vi "LabVIEW to TOML.vi"(8 "error in (no error)":errorcluster, 11 "LV Value":variant) -> (0 "error out":errorcluster, 2 "Name":string, 3 "TOML Value":T1)   [LabVIEW 2020, in "TOML.lvlib"]
uses:
  TOML.lvlib
  TOML Value.ctl
  Value.ctl
  Value Type.ctl
  Key-Value Pair.ctl
  <vilib>/ErrorRing/Error Ring.xnode
  <vilib>/Utility/Data Type/NI_Data Type.lvlib
  <vilib>/JDP Science/JDP Science Common Utilities/JDP Utility.lvlib
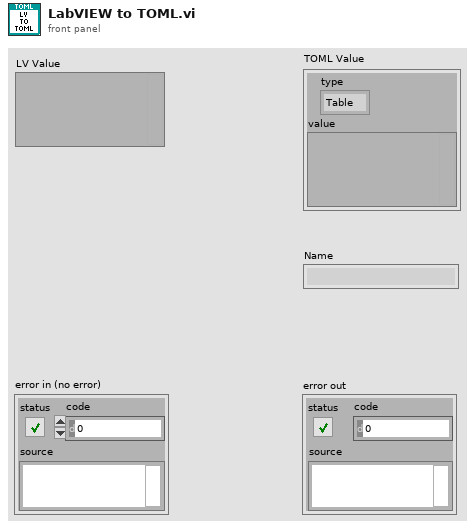
[diagram p1: front panel]
types:
  T1 = typedef "TOML.lvlib/TOML Value.ctl" = cluster{"type":enum16{"Table", "Array", "String", "Integer", "Float", "Boolean", "Offset Date-Time", "Local Date-Time", "Local Date", "Local Time", "Path"}, "value":variant}
  T2 = typedef "TOML.lvlib/Value.ctl" = cluster{"Type":T3, "Value":variant}
  T3 = typedef "TOML.lvlib/Value Type.ctl" = enum16{"Table", "Array", "String", "Integer", "Float", "Boolean", "Offset Date-Time", "Local Date-Time", "Local Date", "Local Time", "Path"}
  T4 = typedef "TOML.lvlib/Key-Value Pair.ctl" = cluster{"Key":string, "Value":T2}
  T5 = typedef "NI_Data Type.lvlib/Data Type.ctl" = enum8{"Invalid Type", "Void", "I8", "I16", "I32", "I64", "U8", "U16", "U32", "U64", "Single Float", "Double Float", "Extended Float", "Single Complex", "Double Complex", "Extended Complex", "Enum U8", "Enum U16", "Enum U32", "Enum U64", "Single Float With Unit", "Double Float With Unit", "Extended Float With Unit", "Single Complex with Unit", "Double Complex with Unit", "Extended Complex with Unit", "Boolean", "String", "Path", "Picture", "Tag", "Array", "Cluster", "Variant", "LV Variant", "Waveform", "Timestamp", "Digital Waveform", "Digital Data", "ExpressData", "Refnum", "External Data", "VI", "Poly VI", "LabVIEW Class Instance", "Fixed Point", "Set Collection", "Map Collection"}
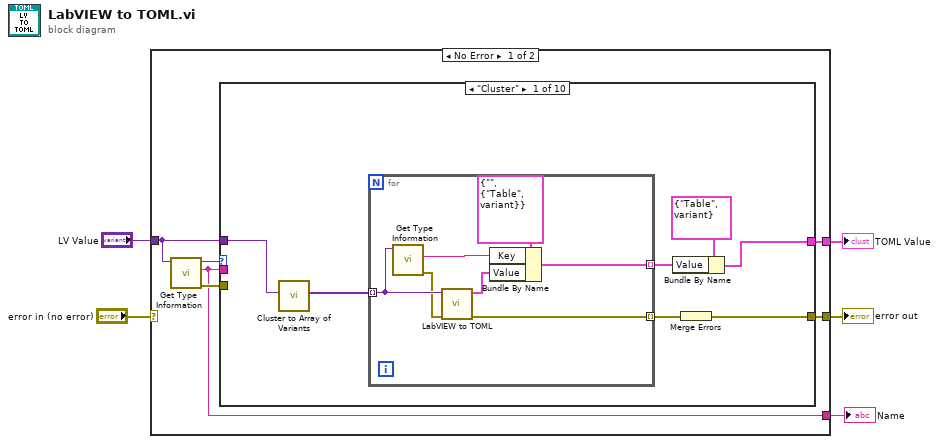
[diagram p0: block diagram]
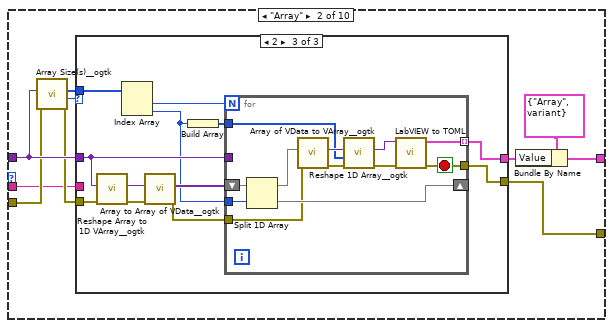
[diagram p2: hidden frame]
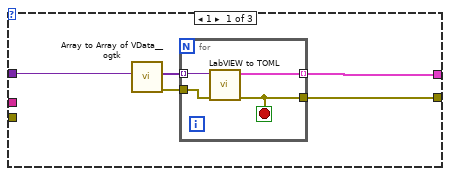
[diagram p3: hidden frame]
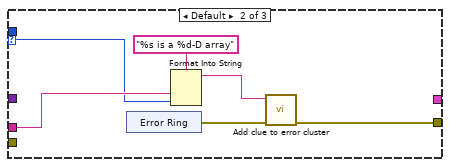
[diagram p4: hidden frame]
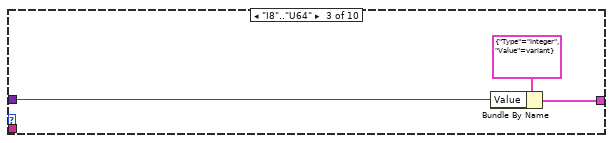
[diagram p5: hidden frame]
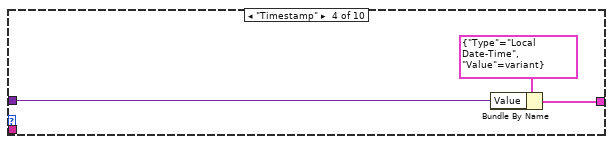
[diagram p6: hidden frame]
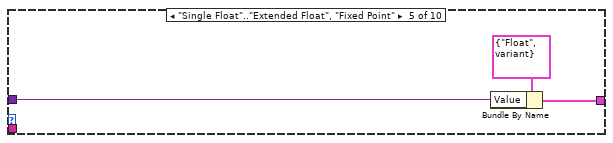
[diagram p7: hidden frame]
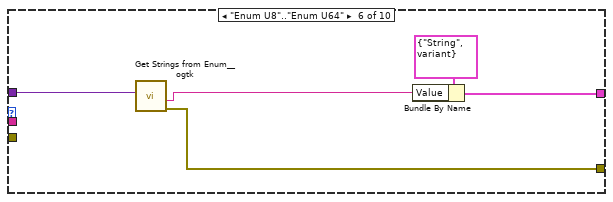
[diagram p8: hidden frame]
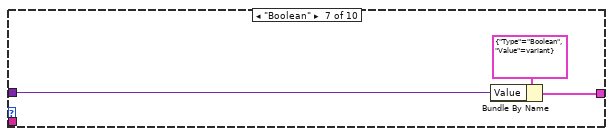
[diagram p9: hidden frame]
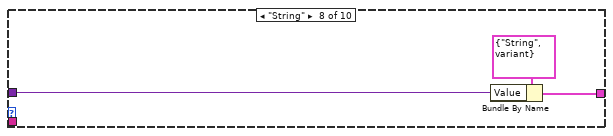
[diagram p10: hidden frame]
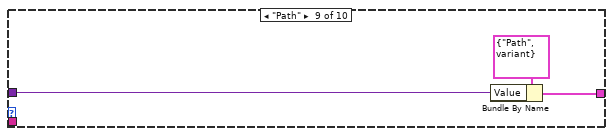
[diagram p11: hidden frame]
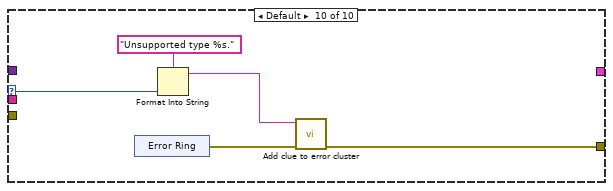
[diagram p12: hidden frame]
diagram:
  n1 = case shown="No Error" "error in (no error)" {
    selector: "error in (no error)" -> [_ w105]
    tunnel: "LV Value" -> [w9 _]
    tunnel: [w10 _] -> w4
    tunnel: [w8 w105] -> w2
    tunnel: [w6 _] -> w1
    frame No Error {
      n2 = call <vilib>:"Get Type Information.vi"("variant"=w9) -> ("error out"=w7:errorcluster, "name"=w6:string, "type"=w11:T5)  [unwired: 6 in, 2 out]
      n3 = case shown="\"Cluster\"" w11 {
        selector: w11 -> [_ _ _ _ _ _ _ _ _ w103]
        tunnel: w9 -> [w16 w35 w76 w79 w82 w89 w90 w93 w96 _]
        tunnel: [w18 w31 w78 w81 w84 w86 w92 w95 w98 _] -> w10
        tunnel: [w17 w29 _ _ _ w85 _ _ _ w100] -> w8
        tunnel: w7 -> [_ w27 _ _ _ _ _ _ _ _]
        tunnel: w6 -> [_ w26 _ _ _ _ _ _ _ _]
        frame "Cluster" {
          n4 = call <vilib>:"Cluster to Array of Variants.vi"("Cluster"=w16) -> ("Array of Cluster Elements"=w15:variant[])  [unwired: 10 in]
          n5 = for {
            tunnel: w15 -> [w25] mode=indexing
            tunnel: [w21] -> w14 mode=indexing
            tunnel: [w19] -> w12 mode=indexing
            n6 = call <vilib>:"Get Type Information.vi"("variant"=w25) -> ("error out"=w20:errorcluster, "name"=w23:string)  [unwired: 6 in, 3 out]
            n7 = call "LabVIEW to TOML.vi"("error in (no error)"=w20, "LV Value"=w25) -> ("error out"=w19:errorcluster, "TOML Value"=w22:T1)  [unwired: 7 in, 1 out]
            n8 = Bundle By Name(cluster=T4 {"Key"="", "Value"={"Type"=enum."Table", "Value"=variant}} ("Key-Value Pair"), "Key"=w23, "Value"=w22) -> (w21:T4)
          }
          n9 = Bundle By Name(cluster=T2 {"Type"=enum."Table", "Value"=variant} ("Value"), "Value"=w14) -> (w18:T2)
          n10 = Merge Errors(w12) -> (w17:errorcluster)
        }
        frame "Array" {
          n11 = call <userlib>:"Array Size(s)__ogtk.vi"("error in (no error)"=w27, "Array"=w35) -> ("error out"=w28:errorcluster, "N dims"=w33:u32, "Size(s)"=w34:u32[])  [unwired: 7 in]
          n12 = case shown="2" w33 {
            selector: w33 -> [_ w45 _]
            tunnel: w35 -> [w40 _ w60]
            tunnel: w34 -> [_ _ w55]
            tunnel: [w38 _ w61] -> w32
            tunnel: [w37 w49 w57] -> w29
            tunnel: w28 -> [_ _ w56]
            tunnel: w26 -> [_ w47 _]
            frame 1 {
              n13 = call <userlib>:"Array to Array of VData__ogtk.vi"("MultiD Array"=w40) -> ("error out"=w36:errorcluster, "1D Array of Variants"=w39:variant[])  [unwired: 9 in]
              n14 = for {
                tunnel: w39 -> [w44] mode=indexing
                tunnel: [w43] -> w38 mode=indexing
                tunnel: [w41] -> w37
                tunnel: w36 -> [w42]
                stop <- w41 stop-if-true
                n15 = call "LabVIEW to TOML.vi"("error in (no error)"=w42, "LV Value"=w44) -> ("error out"=w41:errorcluster, "TOML Value"=w43:T1)  [unwired: 7 in, 1 out]
              }
            }
            frame Default {
              n16 = xnode "Error Ring"() -> ("error out"=w50:errorcluster)
              n17 = Format Into String(format string="%s is a %d-D array", w47, w45) -> (resulting string=w48:string)  [unwired: 2 in, 1 out]
              n18 = call "Add clue to error cluster.vi"("error in (no error)"=w50, "String"=w48) -> ("error out"=w49:errorcluster)  [unwired: 9 in]
            }
            frame 2 {
              n19 = call <userlib>:"Reshape Array to 1D VArray__ogtk.vi"("error in (no error)"=w56, "MultiD Array"=w60) -> ("error out"=w58:errorcluster, "1D VArray"=w63:variant)  [unwired: 7 in, 1 out]
              n20 = Index Array(array=w55) -> (element #1=w54:u32, element #2=w53:u32)  [unwired: 2 in]
              n21 = call <userlib>:"Array to Array of VData__ogtk.vi"("error in (no error)"=w58, "MultiD Array"=w63) -> ("error out"=w59:errorcluster, "1D Array of Variants"=w62:variant[])  [unwired: 8 in]
              n22 = Build Array(w53) -> (w52:u32[])
              n23 = for {
                N: w54 -> [_]
                tunnel: w60 -> [_]
                shift-right: [w69] -> _
                shift-left: w62 -> [w75]
                tunnel: w53 -> [w74]
                tunnel: [w71] -> w61 mode=indexing
                tunnel: w59 -> [w68]
                tunnel: [w67] -> w57
                tunnel: w52 -> [w64]
                stop <- w67 stop-if-true
                n24 = Split 1D Array(array=w75, index=w74) -> (first subarray=w70:variant[], second subarray=w69:variant[])
                n25 = call <userlib>:"Array of VData to VArray__ogtk.vi"("error in (no error)"=w68, "1D Array of VData"=w70) -> ("error out"=w65:errorcluster, "VArray"=w73:variant)  [unwired: 8 in]
                n26 = call <userlib>:"Reshape 1D Array__ogtk.vi"("error in (no error)"=w65, "Size(s)"=w64, "1D Array"=w73) -> ("error out"=w66:errorcluster, "Reshaped VArray"=w72:variant)  [unwired: 7 in]
                n27 = call "LabVIEW to TOML.vi"("error in (no error)"=w66, "LV Value"=w72) -> ("error out"=w67:errorcluster, "TOML Value"=w71:T1)  [unwired: 7 in, 1 out]
              }
            }
          }
          n28 = Bundle By Name(cluster=T2 {"Type"=enum."Array", "Value"=variant} ("Value"), "Value"=w32) -> (w31:T2)
        }
        frame "I8".."U64" {
          n29 = Bundle By Name(cluster=T2 {"Type"=enum."Integer", "Value"=variant} ("Value"), "Value"=w76) -> (w78:T2)
        }
        frame "Timestamp" {
          n30 = Bundle By Name(cluster=T2 {"Type"=enum."Local Date-Time", "Value"=variant} ("Value"), "Value"=w79) -> (w81:T2)
        }
        frame "Single Float".."Extended Float", "Fixed Point" {
          n31 = Bundle By Name(cluster=T2 {"Type"=enum."Float", "Value"=variant} ("Value"), "Value"=w82) -> (w84:T2)
        }
        frame "Enum U8".."Enum U64" {
          n32 = call <userlib>:"Get Strings from Enum__ogtk.vi"("Enum"=w89) -> ("error out"=w85:errorcluster, "String Value"=w87:string)  [unwired: 7 in, 2 out]
          n33 = Bundle By Name(cluster=T2 {"Type"=enum."String", "Value"=variant} ("Value"), "Value"=w87) -> (w86:T2)
        }
        frame "Boolean" {
          n34 = Bundle By Name(cluster=T2 {"Type"=enum."Boolean", "Value"=variant} ("Value"), "Value"=w90) -> (w92:T2)
        }
        frame "String" {
          n35 = Bundle By Name(cluster=T2 {"Type"=enum."String", "Value"=variant} ("Value"), "Value"=w93) -> (w95:T2)
        }
        frame "Path" {
          n36 = Bundle By Name(cluster=T2 {"Type"=enum."Path", "Value"=variant} ("Value"), "Value"=w96) -> (w98:T2)
        }
        frame Default {
          n37 = xnode "Error Ring"() -> ("error out"=w101:errorcluster)
          n38 = Format Into String(format string="Unsupported type %s.", w103) -> (resulting string=w99:string)  [unwired: 2 in, 1 out]
          n39 = call "Add clue to error cluster.vi"("error in (no error)"=w101, "String"=w99) -> ("error out"=w100:errorcluster)  [unwired: 9 in]
        }
      }
    }
    frame Error {
    }
  }
  "error out" <- w2
  "TOML Value" <- w4
  "Name" <- w1
